vi "FeedbackDecode_displayDecodeOutput.vi"(0 "Input":dbl[](array[numeric])) -> ()   [LabVIEW 2020]
panel:
  out "Flexion":dbl[](array[slide]) scale=0.0..2.0
  out "Extension":dbl[](array[slide])
  # "Thumb\nIntrinsic"
  # "Index\nIntrinsic"
  # "Ring\nIntrinsic"
  # "Little\nIntrinsic"
  # "Wrist\nPitch"
  # "Wrist\nYaw"
  # "Wrist\nRoll"
  # "Thumb"
  # "Index"
  # "Middle"
  # "Ring"
  # "Pinky"
  # "Flexion"
  # "Extension"
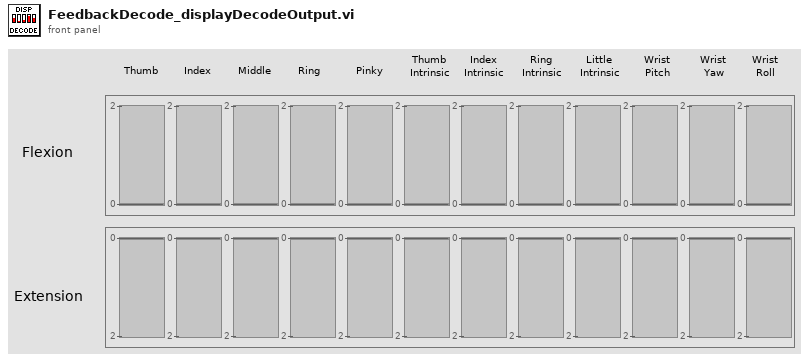
[diagram p1: front panel]
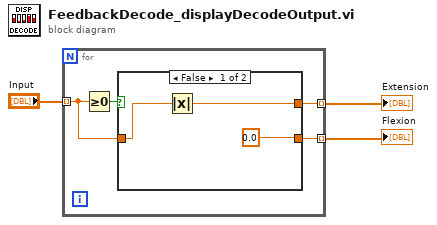
[diagram p0: block diagram]
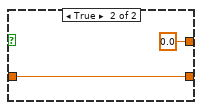
[diagram p2: hidden frame]
diagram:
  n1 = for {
    tunnel: "Input" -> [w6] mode=indexing
    tunnel: [w5] -> w2 mode=indexing
    tunnel: [w4] -> w1 mode=indexing
    n2 = Greater Or Equal To 0?(x=w6) -> (x >= 0?=w7:bool)
    n3 = case shown="False" w7 {
      tunnel: w6 -> [w8 w12]
      tunnel: [0.0 w12] -> w5
      tunnel: [w9 0.0 ("Numeric")] -> w4
      frame False {
        n4 = Absolute Value(x=w8) -> (abs(x)=w9:dbl)
      }
      frame True {
      }
    }
  }
  "Extension" <- w1
  "Flexion" <- w2
